vi "unflatten parameters.vi"(10 "Identifier":string, 11 "Data to Unwrap":string) -> (3 "PID Parameters":T1)   [LabVIEW 2013, in "PID Loop.lvclass"]
uses:
  PID Loop.lvclass
  PID Parameters.ctl
  String Parameters.ctl
  <vilib>/NI/Configuration Framework/serializable configuration/NISE_CEF_serializable configuration.lvclass
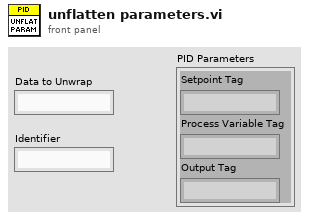
[diagram p1: front panel]
types:
  T1 = typedef "PID Loop.lvclass/PID Parameters.ctl" = cluster{"Setpoint Tag":string, "Process Variable Tag":string, "Output Tag":string}
  T2 = typedef "PID Loop.lvclass/String Parameters.ctl" = enum16{"Setpoint", "Process Variable", "Output", "Proportional Gain", "Integral Time", "Derivative Time", "Range High", "Range Low"}
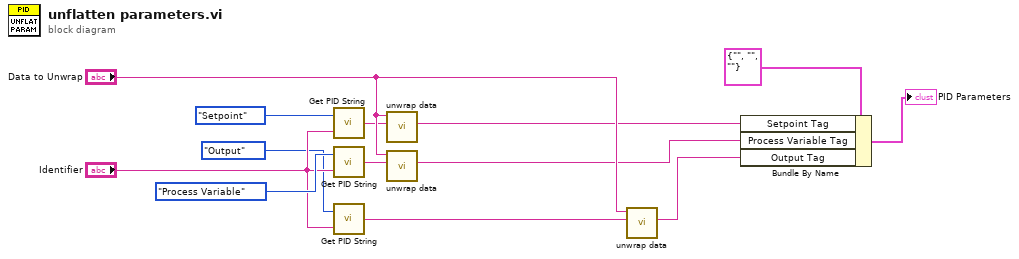
[diagram p0: block diagram]
diagram:
  n1 = call "Get PID String.vi"("PID Loop ID"="Identifier", "PID Parameter"=String_Parameters."Setpoint") -> ("Parameter String"=w2:string)
  n2 = call "Get PID String.vi"("PID Loop ID"="Identifier", "PID Parameter"=String_Parameters."Process Variable") -> ("Parameter String"=w5:string)
  n3 = call "Get PID String.vi"("PID Loop ID"="Identifier", "PID Parameter"=String_Parameters."Output") -> ("Parameter String"=w9:string)
  n4 = call <vilib>:"unwrap data.vi"("identifier"=w2, "data to unwrap"="Data to Unwrap") -> ("unwrapped data"=w4:string)  [unwired: 8 in, 1 out]
  n5 = call <vilib>:"unwrap data.vi"("identifier"=w5, "data to unwrap"="Data to Unwrap") -> ("unwrapped data"=w6:string)  [unwired: 8 in, 1 out]
  n6 = call <vilib>:"unwrap data.vi"("identifier"=w9, "data to unwrap"="Data to Unwrap") -> ("unwrapped data"=w10:string)  [unwired: 8 in, 1 out]
  n7 = Bundle By Name(cluster=T1 {"Setpoint Tag"="", "Process Variable Tag"="", "Output Tag"=""} ("PID Parameters"), "Setpoint Tag"=w4, "Process Variable Tag"=w6, "Output Tag"=w10) -> (→"PID Parameters":T1)
